vi "AutomatedControlDesign.vi"(10 "Output Rate [ticks]":u32, 11 "Sampling Frequency [Hz]":dbl=50000.0 format="%#_13g") -> (0 "K_filt_sos_den":dbl[](array[numeric]), 1 "K_filt_sos_num":dbl[](array[numeric]), 2 "Ki":dbl, 3 "Kp":dbl)   [LabVIEW 2016]
panel:
  in  "Finish":bool
  out "Status Identification":string
  in  "Start Control Design":bool
  in  "Desired closed-loop bandwidth [Hz]":dbl=7000.0 min=500.0 format="%#_13g"
  in  "Start Identification":bool
  out "Frequency Response of Closed-Loop Phase":cluster{dbl[], dbl[]}[](graph)
  out "Frequency Response of Closed-Loop":cluster{dbl[], dbl[]}[](graph)
  out "Frequency Response of Plant Phase":cluster{dbl[], dbl[]}(graph)
  out "Frequency Response of Plant":cluster{dbl[], dbl[]}(graph)
  out "Status Control Design":string
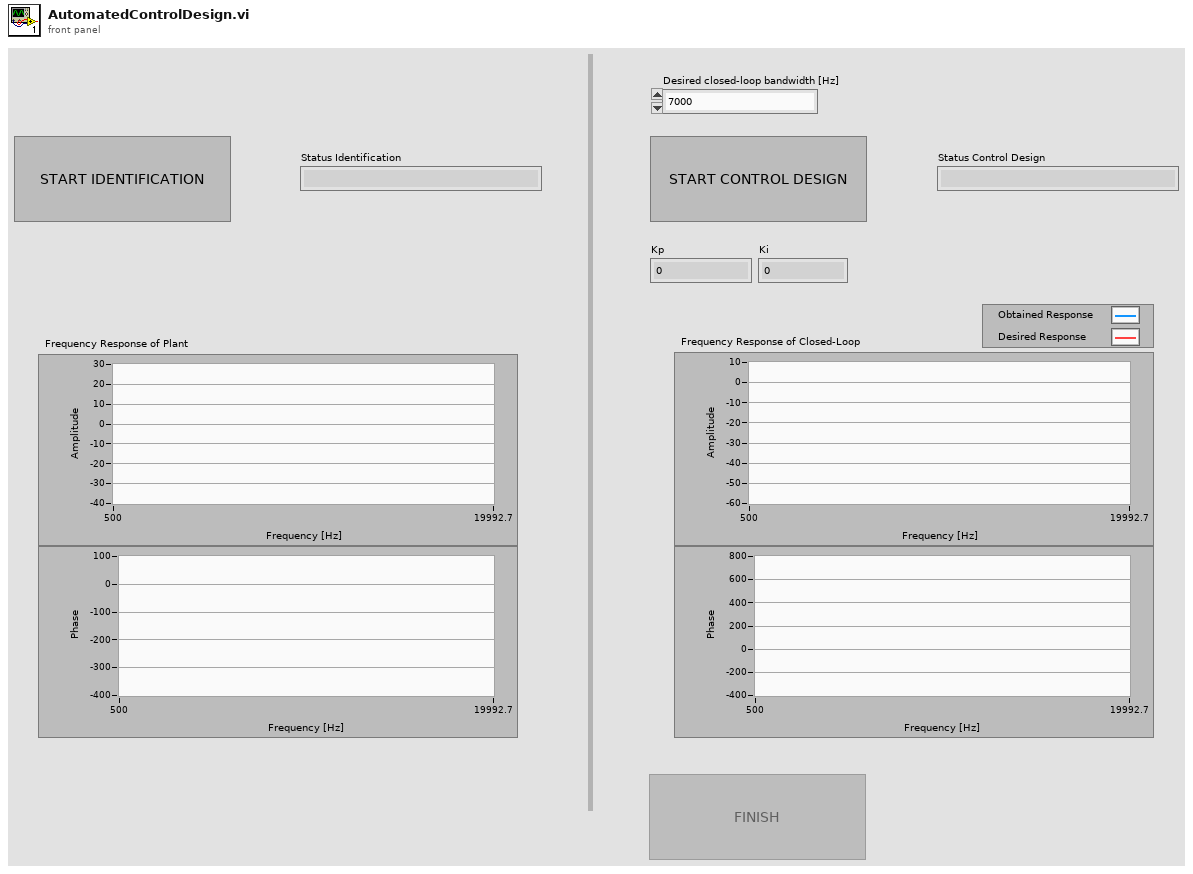
[diagram p1: front panel]
types:
  T1 = enum8{"Enabled", "Disabled", "Disabled and Grayed Out"}
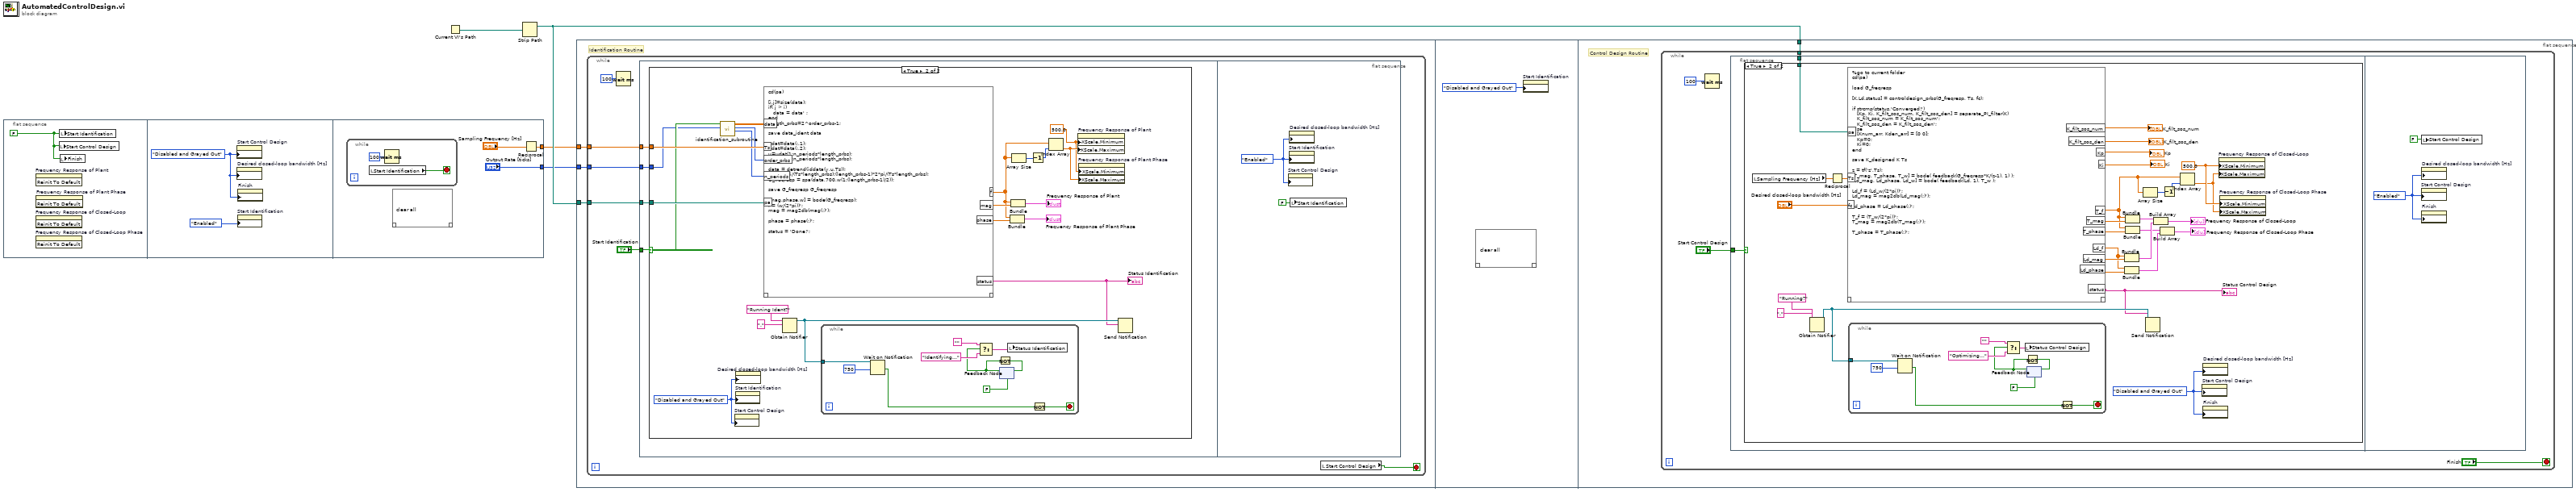
[diagram p0: block diagram]
diagram:
  n1 = flat-sequence {
    tunnel: [w9] -> w2
    tunnel: ["Output Rate [ticks]"] -> w1
    frame #0 {
      w5 = FALSE ("Start Identification")
      n2 = invoke on="Frequency Response of Plant" class="XYGraph (strict)" method="Reinit To Default"() -> ()  [unwired: 3 in, 3 out]
      n3 = invoke on="Frequency Response of Closed-Loop" class="XYGraph (strict)" method="Reinit To Default"() -> ()  [unwired: 3 in, 3 out]
      n4 = invoke on="Frequency Response of Closed-Loop Phase" class="XYGraph (strict)" method="Reinit To Default"() -> ()  [unwired: 3 in, 3 out]
      n5 = invoke on="Frequency Response of Plant Phase" class="XYGraph (strict)" method="Reinit To Default"() -> ()  [unwired: 3 in, 3 out]
      n6 = local write "Start Control Design"(w5) -> ()
      n7 = local write "Start Identification"(w5) -> ()
      n8 = local write "Finish"(w5) -> ()
    }
    frame #1 {
      w6 = T1."Disabled and Grayed Out" ("Disabled")
      n9 = property on="Start Control Design" class="Bool (strict)"("DisabledEnum"=w6) -> ()  [unwired: 2 in, 2 out]
      n10 = property on="Desired closed-loop bandwidth [Hz]" class="DigNum (strict)"("DisabledEnum"=w6) -> ()  [unwired: 2 in, 2 out]
      n11 = property on="Start Identification" class="Bool (strict)"("DisabledEnum"=T1."Enabled" ("Disabled")) -> ()  [unwired: 2 in, 2 out]
      n12 = property on="Finish" class="Bool (strict)"("DisabledEnum"=w6) -> ()  [unwired: 2 in, 2 out]
    }
    frame #2 {
      n13 = while {
        stop <- w12 stop-if-true
        n14 = local read "Start Identification"() -> (w12:bool)
        n15 = Wait (ms)(milliseconds to wait=u32 100) -> ()  [unwired: 1 out]
      }
      n16 = script code="clear all"() -> ()  [unwired: 1 in, 1 out]
      n17 = Reciprocal(x="Sampling Frequency [Hz]") -> (1/x=w9:dbl)
    }
  }
  n18 = Current VI's Path() -> (path=w4:path)
  n19 = Strip Path(path=w4) -> (stripped path=w3:path)  [unwired: 1 out]
  n20 = flat-sequence {
    tunnel: w2 -> [w15]
    tunnel: w3 -> [w14]
    tunnel: w1 -> [w13]
    tunnel: w3 -> [w60]
    frame #0 {
      # "Identification Routine"
      n21 = while {
        tunnel: w15 -> [w21]
        tunnel: w14 -> [w20]
        tunnel: w13 -> [w16]
        stop <- w17 stop-if-true
        n22 = Wait (ms)(milliseconds to wait=u32 100) -> ()  [unwired: 1 out]
        n23 = flat-sequence {
          tunnel: w21 -> [w25]
          tunnel: w20 -> [w24]
          tunnel: "Start Identification" -> [w23]
          tunnel: w16 -> [w22]
          frame #0 {
            n24 = case shown="True" w23 {
              selector: w23 -> [_ w30]
              tunnel: w25 -> [_ w46]
              tunnel: w24 -> [_ w41]
              tunnel: w22 -> [_ w27]
              frame False {
              }
              frame True {
                w31 = T1."Disabled and Grayed Out" ("Disabled")
                w32 = 500.0
                n25 = call "identification_subroutine.vi"("OutputRate"=w27, "Ident Go"=w30) -> ("n_periods"=w28:u16, "order_prbs"=w29:i8, "identdata"=w26:dbl[][])  [unwired: 7 in]
                n26 = property on="Start Control Design" class="Bool (strict)"("DisabledEnum"=w31) -> ()  [unwired: 2 in, 2 out]
                n27 = property on="Start Identification" class="Bool (strict)"("DisabledEnum"=w31) -> ()  [unwired: 2 in, 2 out]
                n28 = property on="Desired closed-loop bandwidth [Hz]" class="DigNum (strict)"("DisabledEnum"=w31) -> ()  [unwired: 2 in, 2 out]
                n29 = script code="cd(pa)\n\n[i,j]=size(data);\nif( j > i)\n   data = data' ;\nend\nlength_prbs=2^order_prbs-1;\n\nsave data_ident data\n\nudat=data(:,1);\nydat=data(:,2);\nu=udat(1:n_periods*length_prbs);\ny=ydat(1:n_periods*length_prbs);\n\ndata = detrend(iddata(y,u,Ts));\nw=0:2*pi/(Ts*length_prbs):(length_prbs-1)*2*pi/(Ts*length_prbs);\nG_freqresp = spa(data,700,w(1:(length_prbs-1)/2));\n\nsave G_freqresp G_freqresp\n\n[mag,phase,w] = bode(G_freqresp);\nf = (w/(2*pi))';\nmag = mag2db(mag(:)');\n\nphase = phase(:)';\n\nstatus = 'Done!';"("Ts"=w46, "n_periods"=w28, "order_prbs"=w29, "pa"=w41, "data"=w26) -> ("mag"=w45:dbl[], "phase"=w44:dbl[], "f"=w36:dbl[], "status"=w37:string)  [unwired: 1 in, 1 out]
                "Status Identification" <- w37
                n30 = Obtain Notifier(name (unnamed)="Running Ident?", notification data type=".") -> (notifier out=w39:refnum<notifier>)  [unwired: 2 in, 2 out]
                n31 = while {
                  tunnel: w39 -> [w56]
                  stop <- w53 stop-if-true
                  n32 = Wait on Notification(notifier=w56, timeout in ms (-1)=750) -> (timed out?=w54:bool)  [unwired: 2 in, 3 out]
                  n33 = feedback #1(FALSE) -> (w49:bool)
                  n34 = Select(t="", s=w49, f="Identifying...") -> (s? t:f=w47:string)
                  n35 = Not(x=w49) -> (.not. x?=w48:bool)
                  n36 = feedback-in #1(w48) -> ()
                  n37 = local write "Status Identification"(w47) -> ()
                  n38 = Not(x=w54) -> (.not. x?=w53:bool)
                }
                n39 = Bundle(w36, w44) -> (→"Frequency Response of Plant Phase":cluster{dbl[], dbl[]})  [unwired: 1 in]
                n40 = Bundle(w36, w45) -> (→"Frequency Response of Plant":cluster{dbl[], dbl[]})  [unwired: 1 in]
                n41 = Array Size(array=w36) -> (size(s)=w35:i32)
                n42 = Decrement(x=w35) -> (x-1=w34:i32)
                n43 = Index Array(array=w36, index=w34) -> (element=w33:dbl)
                n44 = property on="Frequency Response of Plant" class="XYGraph (strict)"("XScale.Minimum"=w32, "XScale.Maximum"=w33) -> ()  [unwired: 2 in, 2 out]
                n45 = property on="Frequency Response of Plant Phase" class="XYGraph (strict)"("XScale.Minimum"=w32, "XScale.Maximum"=w33) -> ()  [unwired: 2 in, 2 out]
                n46 = Send Notification(notification=w37, notifier=w39) -> ()  [unwired: 1 in, 2 out]
              }
            }
          }
          frame #1 {
            w58 = T1."Enabled" ("Disabled")
            n47 = property on="Start Control Design" class="Bool (strict)"("DisabledEnum"=w58) -> ()  [unwired: 2 in, 2 out]
            n48 = property on="Start Identification" class="Bool (strict)"("DisabledEnum"=w58) -> ()  [unwired: 2 in, 2 out]
            n49 = property on="Desired closed-loop bandwidth [Hz]" class="DigNum (strict)"("DisabledEnum"=w58) -> ()  [unwired: 2 in, 2 out]
            n50 = local write "Start Identification"(FALSE ("Start Identification")) -> ()
          }
        }
        n51 = local read "Start Control Design"() -> (w17:bool)
      }
    }
    frame #1 {
      n52 = script code="clear all"() -> ()  [unwired: 1 in, 1 out]
      n53 = property on="Start Identification" class="Bool (strict)"("DisabledEnum"=T1."Disabled and Grayed Out" ("Disabled")) -> ()  [unwired: 2 in, 2 out]
    }
    frame #2 {
      # "Control Design Routine"
      n54 = while {
        tunnel: w60 -> [w64]
        stop <- "Finish" stop-if-true
        n55 = Wait (ms)(milliseconds to wait=u32 100) -> ()  [unwired: 1 out]
        n56 = flat-sequence {
          tunnel: w64 -> [w66]
          tunnel: "Start Control Design" -> [w65]
          frame #0 {
            n57 = case shown="True" w65 {
              tunnel: w66 -> [_ w92]
              frame False {
              }
              frame True {
                w69 = T1."Disabled and Grayed Out" ("Disabled")
                w82 = 500.0
                n58 = local read "Sampling Frequency [Hz]"() -> (w68:dbl)
                n59 = Obtain Notifier(name (unnamed)="Running?", notification data type=".") -> (notifier out=w94:refnum<notifier>)  [unwired: 2 in, 2 out]
                n60 = Reciprocal(x=w68) -> (1/x=w67:dbl)
                n61 = script code="%go to current folder\ncd(pa)\n\nload G_freqresp\n\n[K,Ld,status] = controldesign_prbs(G_freqresp, Ts, fc);\n\nif strcmp(status,'Converged!')\n   [Kp, Ki, K_filt_sos_num, K_filt_sos_den] = separate_PI_filter(K)  \n   K_filt_sos_num = K_filt_sos_num';\n   K_filt_sos_den = K_filt_sos_den';\nelse \n   [Knum_arr, Kden_arr] = [0 0];\n   Kp=0;\n   Ki=0;\nend\n\nsave K_designed K Ts\n\nz = tf('z',Ts);\n[T_mag, T_phase, T_w] = bode( feedback(G_freqresp*K/(z-1), 1) );\n[Ld_mag, Ld_phase, Ld_w] = bode( feedback(Ld, 1), T_w );\n\nLd_f = (Ld_w/(2*pi))';\nLd_mag = mag2db(Ld_mag(:)');\n\nLd_phase = Ld_phase(:)';\n\nT_f = (T_w/(2*pi))';\nT_mag = mag2db(T_mag(:)');\n\nT_phase = T_phase(:)';"("pa"=w92, "fc"="Desired closed-loop bandwidth [Hz]", "Ts"=w67) -> ("K_filt_sos_num"=→"K_filt_sos_num":dbl[], "K_filt_sos_den"=→"K_filt_sos_den":dbl[], "status"=w76:string, "Kp"=→"Kp":dbl, "Ki"=→"Ki":dbl, "T_mag"=w91:dbl[], "T_phase"=w90:dbl[], "T_f"=w75:dbl[], "Ld_f"=w88:dbl[], "Ld_mag"=w89:dbl[], "Ld_phase"=w87:dbl[])  [unwired: 1 in, 1 out]
                "Status Control Design" <- w76
                n62 = while {
                  tunnel: w94 -> [w105]
                  stop <- w102 stop-if-true
                  n63 = Wait on Notification(notifier=w105, timeout in ms (-1)=750) -> (timed out?=w103:bool)  [unwired: 2 in, 3 out]
                  n64 = feedback #2(FALSE) -> (w97:bool)
                  n65 = Select(t="", s=w97, f="Optimizing...") -> (s? t:f=w99:string)
                  n66 = local write "Status Control Design"(w99) -> ()
                  n67 = Not(x=w97) -> (.not. x?=w96:bool)
                  n68 = feedback-in #2(w96) -> ()
                  n69 = Not(x=w103) -> (.not. x?=w102:bool)
                }
                n70 = Bundle(w88, w89) -> (w85:cluster{dbl[], dbl[]})  [unwired: 1 in]
                n71 = Bundle(w88, w87) -> (w83:cluster{dbl[], dbl[]})  [unwired: 1 in]
                n72 = Bundle(w75, w91) -> (w86:cluster{dbl[], dbl[]})  [unwired: 1 in]
                n73 = Bundle(w75, w90) -> (w84:cluster{dbl[], dbl[]})  [unwired: 1 in]
                n74 = Array Size(array=w75) -> (size(s)=w79:i32)
                n75 = Send Notification(notification=w76, notifier=w94) -> ()  [unwired: 1 in, 2 out]
                n76 = Build Array(w86, w85) -> (→"Frequency Response of Closed-Loop":cluster{dbl[], dbl[]}[])
                n77 = Build Array(w84, w83) -> (→"Frequency Response of Closed-Loop Phase":cluster{dbl[], dbl[]}[])
                n78 = Decrement(x=w79) -> (x-1=w80:i32)
                n79 = Index Array(array=w75, index=w80) -> (element=w81:dbl)
                n80 = property on="Start Control Design" class="Bool (strict)"("DisabledEnum"=w69) -> ()  [unwired: 2 in, 2 out]
                n81 = property on="Desired closed-loop bandwidth [Hz]" class="DigNum (strict)"("DisabledEnum"=w69) -> ()  [unwired: 2 in, 2 out]
                n82 = property on="Finish" class="Bool (strict)"("DisabledEnum"=w69) -> ()  [unwired: 2 in, 2 out]
                n83 = property on="Frequency Response of Closed-Loop" class="XYGraph (strict)"("XScale.Minimum"=w82, "XScale.Maximum"=w81) -> ()  [unwired: 2 in, 2 out]
                n84 = property on="Frequency Response of Closed-Loop Phase" class="XYGraph (strict)"("XScale.Minimum"=w82, "XScale.Maximum"=w81) -> ()  [unwired: 2 in, 2 out]
              }
            }
          }
          frame #1 {
            w106 = T1."Enabled" ("Disabled")
            n85 = local write "Start Control Design"(FALSE ("Start Control Design")) -> ()
            n86 = property on="Start Control Design" class="Bool (strict)"("DisabledEnum"=w106) -> ()  [unwired: 2 in, 2 out]
            n87 = property on="Desired closed-loop bandwidth [Hz]" class="DigNum (strict)"("DisabledEnum"=w106) -> ()  [unwired: 2 in, 2 out]
            n88 = property on="Finish" class="Bool (strict)"("DisabledEnum"=w106) -> ()  [unwired: 2 in, 2 out]
          }
        }
      }
    }
  }
